vi "TroncateGraphData.vi"(0 "TimeStampTreshold":dbl format="%.3f", 7 "Data IN":cluster{dbl[], dbl[]}[](array[cluster]) {"?" format="%.3f"}) -> (8 "Truncated Data":cluster{dbl[], dbl[]}[](array[cluster]) {"?" format="%.3f"})   [LabVIEW 2011]
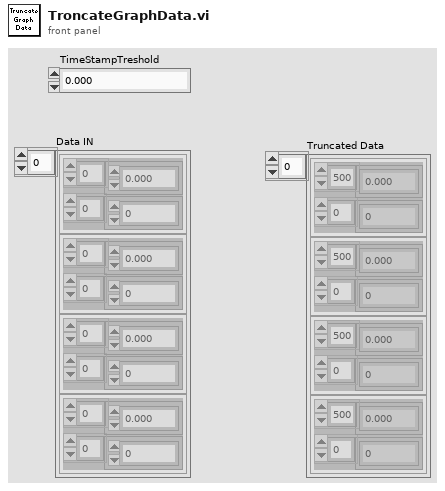
[diagram p1: front panel]
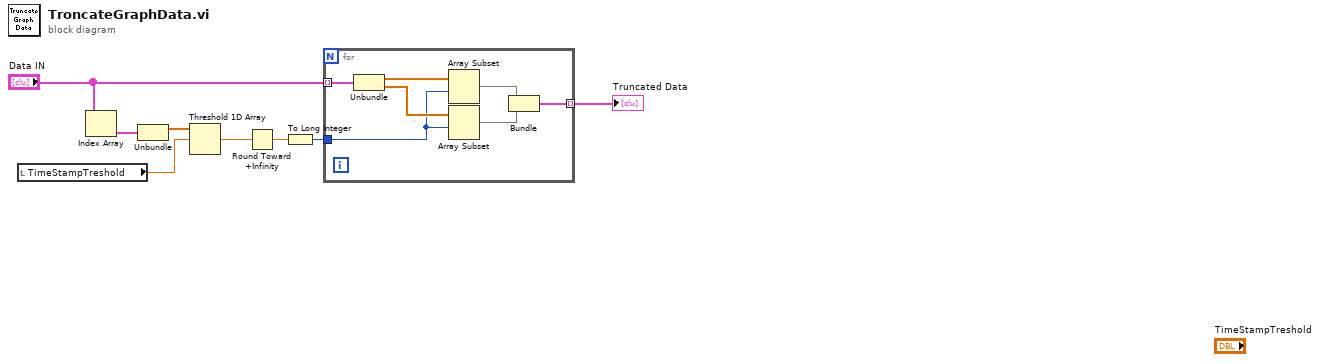
[diagram p0: block diagram]
diagram:
  n1 = local read "TimeStampTreshold"() -> (w5:dbl)
  n2 = Index Array(array="Data IN") -> (element=w7:cluster{dbl[], dbl[]})  [unwired: 1 in]
  n3 = Unbundle(w7) -> (w6:dbl[])  [unwired: 1 out]
  n4 = Threshold 1D Array(2:w5, 3:w6) -> (0:w3:dbl)  [unwired: 1 in]
  n5 = Round Toward +Infinity(x=w3) -> (ceil(x): smallest int >= x=w4:dbl)
  n6 = To Long Integer(number=w4) -> (32bit integer=w2:i32)
  n7 = for {
    tunnel: "Data IN" -> [w15] mode=indexing
    tunnel: w2 -> [w9]
    tunnel: [w10] -> w1 mode=indexing
    n8 = Unbundle(w15) -> (w14:dbl[], w13:dbl[])
    n9 = Array Subset(array=w14, index=w9) -> (w12:dbl[])  [unwired: 1 in]
    n10 = Array Subset(array=w13, index=w9) -> (w11:dbl[])  [unwired: 1 in]
    n11 = Bundle(w12, w11) -> (w10:cluster{dbl[], dbl[]})  [unwired: 1 in]
  }
  "Truncated Data" <- w1
